vi "ryvisa_query.vi"(4 "visa timeout (0=ignore)":u32, 6 "ms read wait (0)":u32, 8 "error in (no error)":errorcluster, 9 "byte count (0=no read)":u32, 10 "write buffer (\"\"=no write)":string, 11 "visa in":refnum<visa-resource-name>) -> (0 "error out":errorcluster, 1 "return count":u32, 2 "read buffer":string, 3 "visa out":refnum<visa-resource-name>)   [LabVIEW 2017]
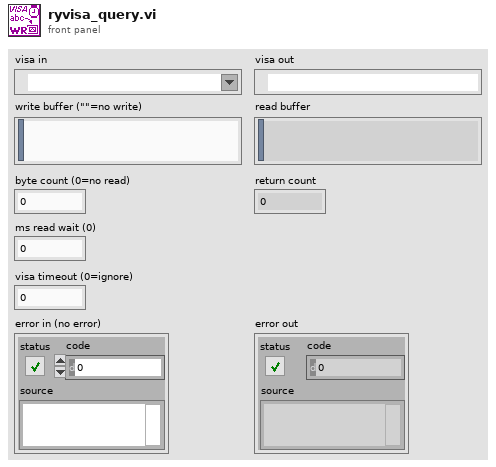
[diagram p1: front panel]
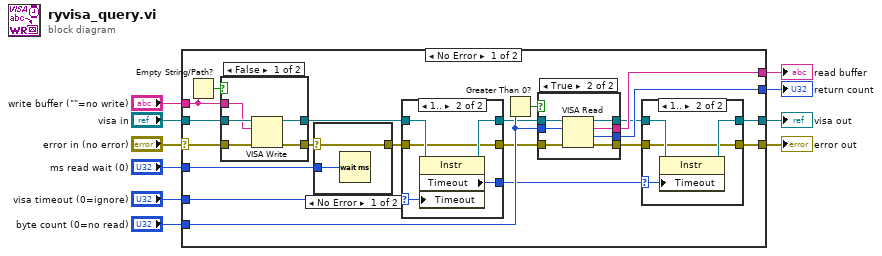
[diagram p0: block diagram]
diagram:
  n1 = case shown="No Error" "error in (no error)" {
    selector: "error in (no error)" -> [w30 w64]
    tunnel: "visa in" -> [w29 w63]
    tunnel: [w28 w64] -> w8
    tunnel: [w27 w63] -> w7
    tunnel: "visa timeout (0=ignore)" -> [w26 _]
    tunnel: "write buffer (\"\"=no write)" -> [w25 _]
    tunnel: "ms read wait (0)" -> [w24 _]
    tunnel: "byte count (0=no read)" -> [w23 _]
    tunnel: [w22 _] -> w2
    tunnel: [w21 _] -> w1
    frame No Error {
      n2 = Empty String/Path?(string/path=w25) -> (empty?=w20:bool)
      n3 = case shown="False" w20 {
        tunnel: w30 -> [w44 w46]
        tunnel: w29 -> [w43 w45]
        tunnel: w25 -> [w41 _]
        tunnel: [w42 w46] -> w18
        tunnel: [w40 w45] -> w17
        frame False {
          n4 = VISA Write(VISA resource name=w43, write buffer=w41, error in (no error)=w44) -> (VISA resource name out=w40:refnum<visa-resource-name>, error out=w42:errorcluster)  [unwired: 1 out]
        }
        frame True {
        }
      }
      n5 = case shown="No Error" w18 {
        tunnel: w24 -> [w32 _]
        tunnel: [w31 w33] -> w19
        selector: w18 -> [w31 w33]
        frame No Error {
          n6 = Wait (ms)(milliseconds to wait=w32) -> ()  [unwired: 1 out]
        }
        frame Error {
        }
      }
      n7 = case shown="1.." w26 {
        selector: w26 -> [_ w61]
        tunnel: [w56 w58] -> w15
        tunnel: [w57 w62] -> w16
        tunnel: w19 -> [w56 w58]
        tunnel: w17 -> [w57 w60]
        tunnel: [_ w59] -> w11
        frame 0 {
        }
        frame 1.. {
          n8 = property class="Instr"(reference=w60, "Timeout"=w61) -> (reference out=w62:refnum<visa-resource-name>, "Timeout"=w59:u32)  [unwired: 1 in, 1 out]
        }
      }
      n9 = Greater Than 0?(x=w23) -> (x > 0?=w14:bool)
      n10 = case shown="True" w14 {
        tunnel: w16 -> [w48 w55]
        tunnel: [w48 w54] -> w13
        tunnel: w15 -> [w47 w53]
        tunnel: [w47 w52] -> w12
        tunnel: w23 -> [_ w51]
        tunnel: [_ w50] -> w22
        tunnel: [_ w49] -> w21
        frame False {
        }
        frame True {
          n11 = VISA Read(VISA resource name=w55, byte count=w51, error in (no error)=w53) -> (VISA resource name out=w54:refnum<visa-resource-name>, read buffer=w50:string, return count=w49:u32, error out=w52:errorcluster)
        }
      }
      n12 = case shown="1.." w11 {
        selector: w11 -> [_ w38]
        tunnel: [w34 w36] -> w28
        tunnel: [w35 w39] -> w27
        tunnel: w12 -> [w34 w36]
        tunnel: w13 -> [w35 w37]
        frame 0 {
        }
        frame 1.. {
          n13 = property class="Instr"(reference=w37, "Timeout"=w38) -> (reference out=w39:refnum<visa-resource-name>)  [unwired: 1 in, 1 out]
        }
      }
    }
    frame Error {
    }
  }
  "error out" <- w8
  "visa out" <- w7
  "read buffer" <- w2
  "return count" <- w1
